vi "Close Tab.vi"(8 "error in":errorcluster, 11 "Tab Control Reference In":refnum<vi>) -> (0 "error out":errorcluster, 3 "Tab Control Reference Out":refnum<vi>)   [LabVIEW 2017, in "DTacq Plot Display Library.lvlib"]
doc: "Prepares the graphical user interface for display;\nGUI controls are set to their default values,\nThe front panel is centered on the screen,\nThe front panel is opened, if not already open"
uses:
  DTacq Plot Display Library.lvlib
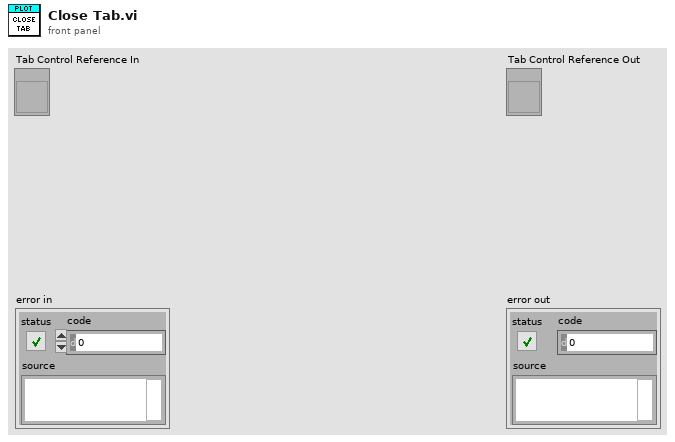
[diagram p1: front panel]
types:
  T1 = enum32{"Page 1", "Page 2", "Page 3", "Page 4", "Page 5", "Page 6"}
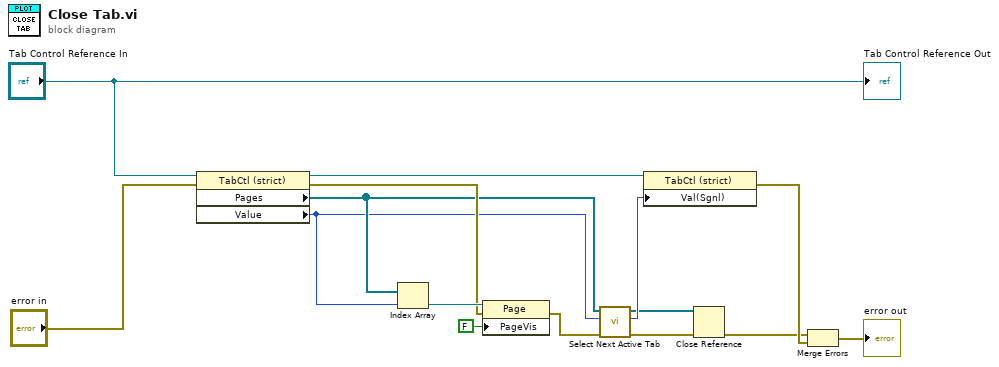
[diagram p0: block diagram]
diagram:
  n1 = property class="TabCtl (strict)"(reference="Tab Control Reference In", error in="error in") -> (reference out=w7:refnum<vi>, error out=w11:errorcluster, "Pages"=w10:refnum<vi>[], "Value"=w8:T1)
  n2 = Index Array(array=w10, index=w8) -> (element=w13:refnum<vi>)
  n3 = property class="Page"(reference=w13, error in=w11, "PageVis"=FALSE ("Page Visible")) -> (error out=w9:errorcluster)  [unwired: 1 out]
  n4 = call "Select Next Active Tab.vi"("error in"=w9, "Current Tab"=w8, "Tab Pages References In"=w10) -> ("error out"=w2:errorcluster, "Next Tab"=w6:i32, "Tab Pages References Out"=w1:refnum<vi>[])  [unwired: 6 in]
  n5 = property class="TabCtl (strict)"(reference=w7, "Val(Sgnl)"=w6) -> (error out=w5:errorcluster)  [unwired: 1 in, 1 out]
  n6 = Close Reference(reference=w1, error in (no error)=w2) -> (error out=w3:errorcluster)
  n7 = Merge Errors(w3, w5) -> (→"error out":errorcluster)
  "Tab Control Reference Out" <- "Tab Control Reference In"
